vi "Solve1.vi"(8 "Error In":errorcluster, 11 "object in":refnum<class "2021_5.lvclass">) -> (0 "Error Out":errorcluster, 2 "Result":u64, 3 "object out":refnum<class "2021_5.lvclass">)   [LabVIEW 2020, in "2021_5.lvclass"]
uses:
  2021_5.lvclass
  2021_5.lvclass/2021_5.ctl
  <vilib>/numeric/Random Number (Range) U64.vi
  <vilib>/numeric/sub_Random U32.vi
panel:
  out "2D Picture":picture
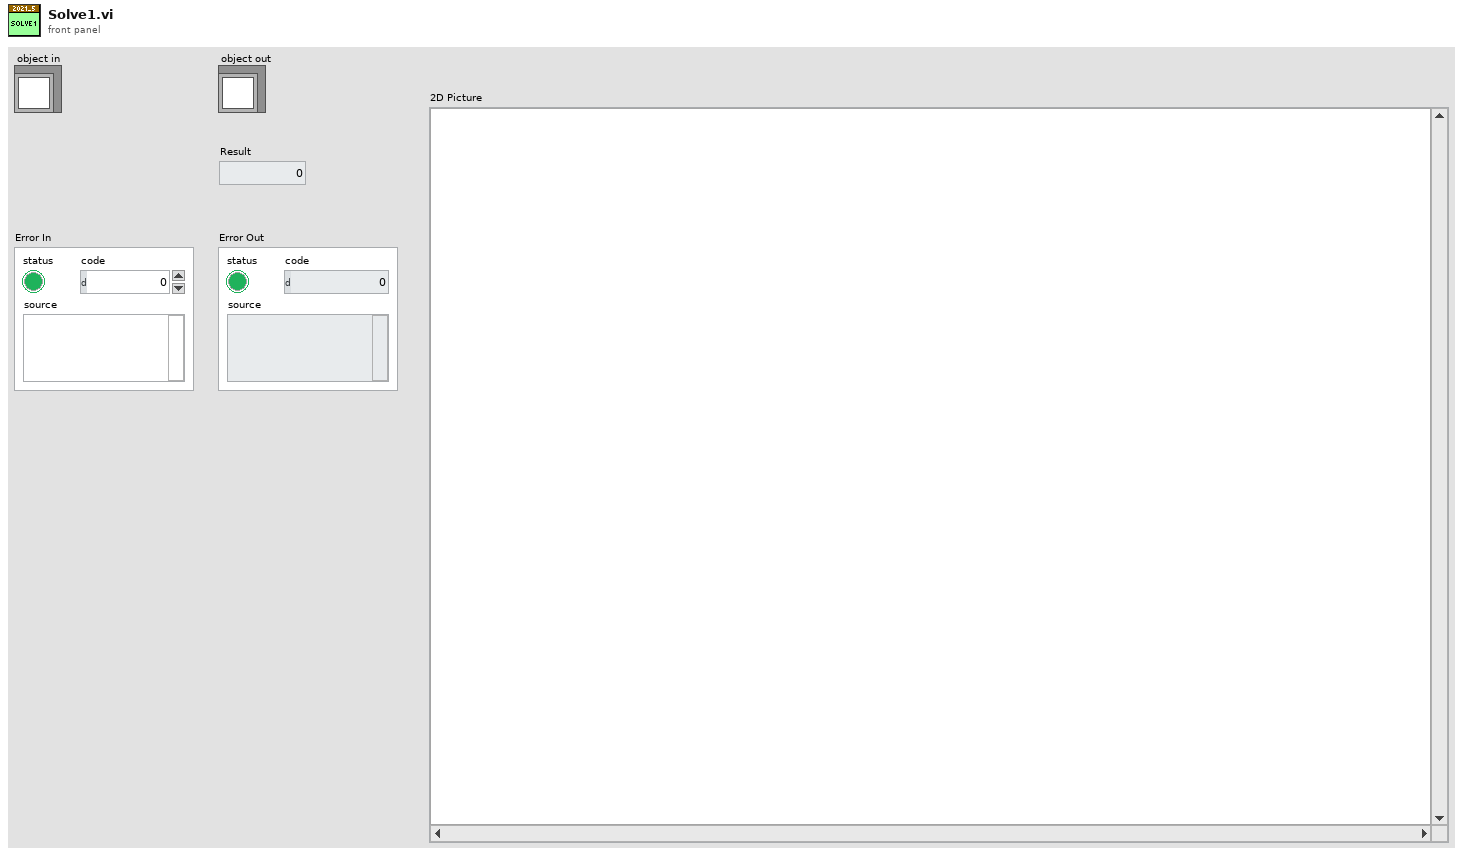
[diagram p1: front panel]
types:
  T1 = cluster{"Point1":cluster{"X":i32, "Y":i32}, "Point2":cluster{"X":i32, "Y":i32}}[]
  T2 = typedef "imagedata.ctl" = cluster{"image type":i32, "image depth":i32, "image":u8[], "mask":u8[], "colors":u32[], "Rectangle":cluster{"left":i16, "top":i16, "right":i16, "bottom":i16}}
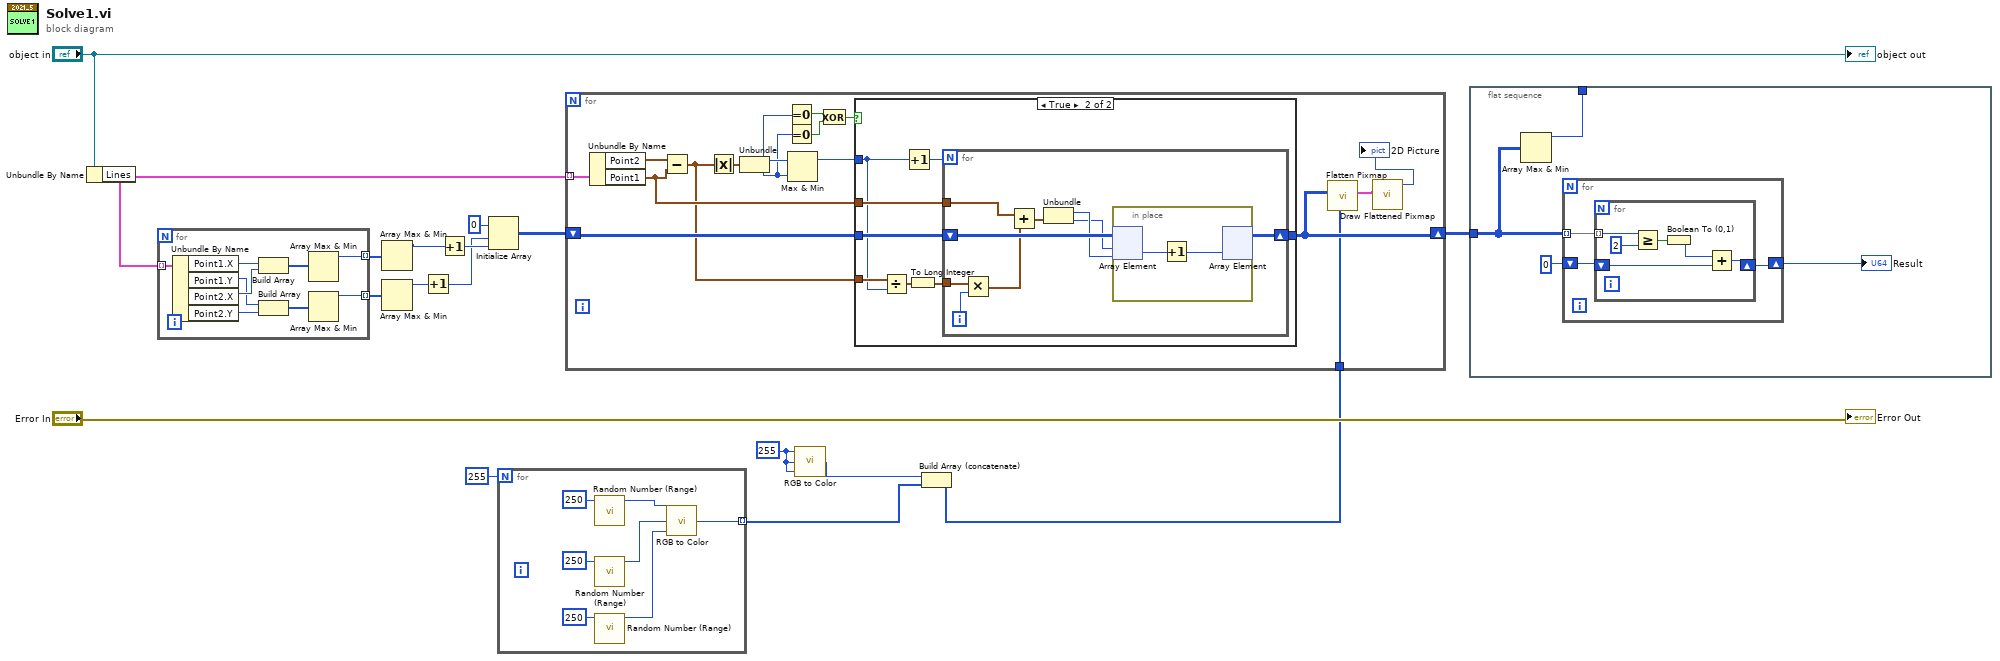
[diagram p0: block diagram]
diagram:
  w4 = 255
  n1 = Unbundle By Name("object in") -> ("Lines"=w15:T1)
  n2 = for {
    tunnel: w15 -> [w26] mode=indexing
    tunnel: [w20] -> w13 mode=indexing
    tunnel: [w18] -> w14 mode=indexing
    n3 = Unbundle By Name(w26) -> ("Point1.X"=w25:i32, "Point1.Y"=w22:i32, "Point2.X"=w24:i32, "Point2.Y"=w23:i32)
    n4 = Build Array(w25, w24) -> (w21:i32[])
    n5 = Build Array(w22, w23) -> (w19:i32[])
    n6 = Array Max & Min(array=w21) -> (max value=w20:i32)  [unwired: 3 out]
    n7 = Array Max & Min(array=w19) -> (max value=w18:i32)  [unwired: 3 out]
  }
  n8 = Array Max & Min(array=w13) -> (max value=w11:i32)  [unwired: 3 out]
  n9 = Array Max & Min(array=w14) -> (max value=w12:i32)  [unwired: 3 out]
  n10 = Increment(x=w12) -> (x+1=w7:i32)
  n11 = Increment(x=w11) -> (x+1=w8:i32)
  n12 = Initialize Array(u32 0 ("length"), w7, w8) -> (w9:u32[][])
  n13 = for {
    N: 255 -> [_]
    tunnel: [w33] -> w2 mode=indexing
    n14 = call-poly <vilib>:"Random Number (Range).vi"("upper bound (100)"=u64 250) -> ("number"=w29:u64)  [unwired: 10 in]
    n15 = call-poly <vilib>:"Random Number (Range).vi"("upper bound (100)"=u64 250) -> ("number"=w28:u64)  [unwired: 10 in]
    n16 = call-poly <vilib>:"Random Number (Range).vi"("upper bound (100)"=u64 250) -> ("number"=w27:u64)  [unwired: 10 in]
    n17 = call <vilib>:"RGB to Color.vi"("B"=w27, "G"=w28, "R"=w29) -> ("Color"=w33:u32)
  }
  n18 = call <vilib>:"RGB to Color.vi"("B"=w4, "G"=w4, "R"=w4) -> ("Color"=w3:u32)
  n19 = Build Array (concatenate)(w3, w2) -> (w1:u32[])
  n20 = for {
    tunnel: w15 -> [w49] mode=indexing
    shift-right: [w42] -> w6
    shift-left: w9 -> [w47]
    tunnel: w1 -> [w39]
    n21 = Unbundle By Name(w49) -> ("Point2"=w48:cluster{"X":i32, "Y":i32}, "Point1"=w46:cluster{"X":i32, "Y":i32})
    n22 = Subtract(x=w48, y=w46) -> (x-y=w44:cluster{"X":i32, "Y":i32})
    n23 = Absolute Value(x=w44) -> (abs(x)=w45:cluster{"X":i32, "Y":i32})
    n24 = Unbundle(w45) -> ("X"=w38:i32, "Y"=w37:i32)
    n25 = Equal To 0?(x=w38) -> (x = 0?=w36:bool)
    n26 = Equal To 0?(x=w37) -> (x = 0?=w35:bool)
    n27 = Max & Min(x=w38, y=w37) -> (max(x,y)=w43:i32)  [unwired: 1 out]
    n28 = Exclusive Or(1:w35, 2:w36) -> (0:w34:bool)
    n29 = case shown="True" w34 {
      tunnel: w47 -> [w50 w58]
      tunnel: w46 -> [_ w57]
      tunnel: w44 -> [_ w55]
      tunnel: w43 -> [_ w54]
      tunnel: [w50 w52] -> w42
      frame False {
      }
      frame True {
        n30 = Divide(x=w55, y=w54) -> (x/y=w53:cluster{"X":dbl, "Y":dbl})
        n31 = Increment(x=w54) -> (x+1=w56:i32)
        n32 = To Long Integer(number=w53) -> (32bit integer=w51:cluster{"X":i32, "Y":i32})
        n33 = for {
          N: w56 -> [_]
          shift-right: [w66] -> w52
          shift-left: w58 -> [w67]
          tunnel: w57 -> [w63]
          tunnel: w51 -> [w59]
          i -> [w61]
          n34 = Multiply(x=w59, y=w61) -> (x*y=w60:cluster{"X":i32, "Y":i32})
          n35 = Add(x=w63, y=w60) -> (x+y=w62:cluster{"X":i32, "Y":i32})
          n36 = Unbundle(w62) -> ("X"=w65:i32, "Y"=w64:i32)
          n37 = in-place {
            n38 = in-place-array #1(w67, w64, w65) -> (w69:u32)
            n39 = Increment(x=w69) -> (x+1=w68:u32)
            n40 = in-place-array #1(w68) -> (w66:u32[][])  [unwired: 2 out]
          }
        }
      }
    }
    n41 = call <vilib>:"Flatten Pixmap.vi"("colors"=w39, "8-bit pixmap"=w42) -> ("image data"=w41:T2)  [unwired: 9 in]
    n42 = call <vilib>:"Draw Flattened Pixmap.vi"("image data"=w41) -> ("new picture"=→"2D Picture":picture)  [unwired: 8 in]
  }
  n43 = flat-sequence {
    tunnel: w6 -> [w71]
    tunnel: [w70] -> _
    frame #0 {
      n44 = Array Max & Min(array=w71) -> (max value=w70:u32)  [unwired: 3 out]
      n45 = for {
        tunnel: w71 -> [w76] mode=indexing
        shift-right: [w74] -> w72
        shift-left: u32 0 ("length") -> [w75]
        n46 = for {
          tunnel: w76 -> [w82] mode=indexing
          shift-right: [w77] -> w74
          shift-left: w75 -> [w79]
          n47 = Greater Or Equal?(x=w82, y=u32 2) -> (x >= y?=w80:bool)
          n48 = Boolean To (0,1)(Boolean=w80) -> (0, 1=w78:i16)
          n49 = Add(x=w78, y=w79) -> (x+y=w77:u32)
        }
      }
      "Result" <- w72
    }
  }
  "Error Out" <- "Error In"
  "object out" <- "object in"
